vi "Test Assert Almost Equal (Float).vi"(8 "error in (no error)":errorcluster) -> (0 "error out":errorcluster)   [LabVIEW 2020]
uses:
  classes/Assert/Assert.lvclass
  classes/Test/Test.lvclass
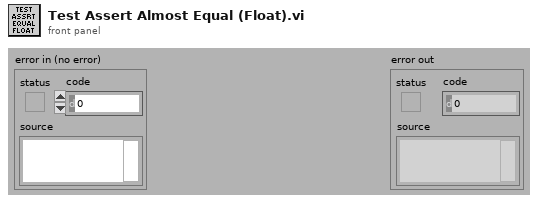
[diagram p1: front panel]
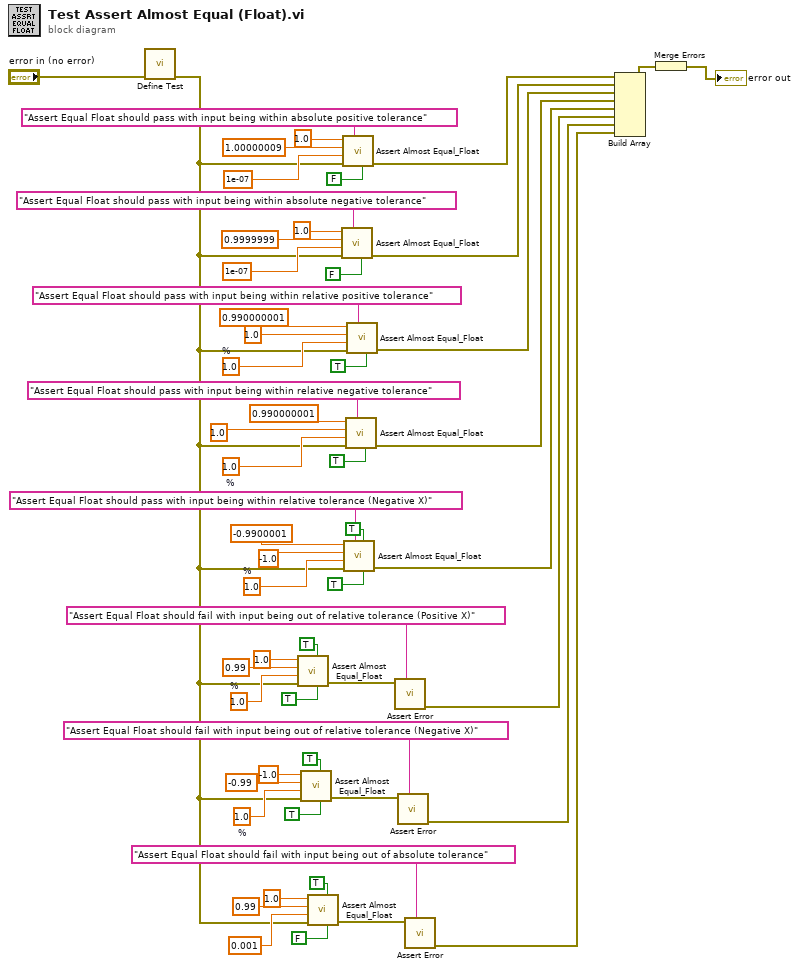
[diagram p0: block diagram]
diagram:
  w13 = 1.0  # %
  w19 = 1.0  # %
  w32 = 1.0  # %
  w39 = 1.0  # %
  w42 = 1.0  # %
  n1 = call "Define Test.vi"("error in (no error)"="error in (no error)") -> ("error out"=w7:errorcluster)  [unwired: 9 in, 1 out]
  n2 = call "Assert Almost Equal_Float.vi"("Use Percentage of X (F)"=TRUE, "Assert Only? (F)"=TRUE, "error in (no error)"=w7, "Tolerance"=w32, "Y"=0.99, "X"=1.0) -> ("error out"=w30:errorcluster)  [unwired: 4 in, 1 out]
  n3 = call "Assert Almost Equal_Float.vi"("Use Percentage of X (F)"=TRUE, "Assert Only? (F)"=TRUE, "error in (no error)"=w7, "Tolerance"=w13, "Y"=-0.99, "X"=-1.0) -> ("error out"=w15:errorcluster)  [unwired: 4 in, 1 out]
  n4 = call "Assert Almost Equal_Float.vi"("Use Percentage of X (F)"=FALSE, "Assert Only? (F)"=TRUE, "error in (no error)"=w7, "Tolerance"=0.001, "Y"=0.99, "X"=1.0) -> ("error out"=w28:errorcluster)  [unwired: 4 in, 1 out]
  n5 = call "Assert Almost Equal_Float.vi"("Use Percentage of X (F)"=FALSE, "Label"="Assert Equal Float should pass with input being within absolute negative tolerance", "error in (no error)"=w7, "Tolerance"=1e-07, "Y"=0.9999999, "X"=1.0) -> ("error out"=w45:errorcluster)  [unwired: 4 in, 1 out]
  n6 = call "Assert Almost Equal_Float.vi"("Use Percentage of X (F)"=FALSE, "Label"="Assert Equal Float should pass with input being within absolute positive tolerance", "error in (no error)"=w7, "Tolerance"=1e-07, "Y"=1.00000009, "X"=1.0) -> ("error out"=w55:errorcluster)  [unwired: 4 in, 1 out]
  n7 = call "Assert Almost Equal_Float.vi"("Use Percentage of X (F)"=TRUE, "Assert Only? (F)"=TRUE, "Label"="Assert Equal Float should pass with input being within relative tolerance (Negative X)", "error in (no error)"=w7, "Tolerance"=w19, "Y"=-1.0, "X"=-0.9900001) -> ("error out"=w16:errorcluster)  [unwired: 3 in, 1 out]
  n8 = call "Assert Almost Equal_Float.vi"("Use Percentage of X (F)"=TRUE, "Label"="Assert Equal Float should pass with input being within relative negative tolerance", "error in (no error)"=w7, "Tolerance"=w39, "Y"=1.0, "X"=0.990000001) -> ("error out"=w37:errorcluster)  [unwired: 4 in, 1 out]
  n9 = call "Assert Almost Equal_Float.vi"("Use Percentage of X (F)"=TRUE, "Label"="Assert Equal Float should pass with input being within relative positive tolerance", "error in (no error)"=w7, "Tolerance"=w42, "Y"=1.0, "X"=0.990000001) -> ("error out"=w38:errorcluster)  [unwired: 4 in, 1 out]
  n10 = call "Assert Error.vi"("Label"="Assert Equal Float should fail with input being out of relative tolerance (Positive X)", "Error?"=w30) -> ("error out"=w29:errorcluster)  [unwired: 8 in, 1 out]
  n11 = call "Assert Error.vi"("Label"="Assert Equal Float should fail with input being out of relative tolerance (Negative X)", "Error?"=w15) -> ("error out"=w8:errorcluster)  [unwired: 8 in, 1 out]
  n12 = call "Assert Error.vi"("Label"="Assert Equal Float should fail with input being out of absolute tolerance", "Error?"=w28) -> ("error out"=w21:errorcluster)  [unwired: 8 in, 1 out]
  n13 = Build Array(w55, w45, w38, w37, w16, w29, w8, w21) -> (w57:errorcluster[])
  n14 = Merge Errors(w57) -> (→"error out":errorcluster)
